vi "PWM Waveform Generator.vi"(4 "Compare Output Mode":fxp<+,2,2> format="%02b", 5 "Enable In":bool, 6 "Waveform Generation Mode":fxp<+,2,2> format="%02b", 7 "Counter is Output Compare?":bool, 10 "Counter is Min?":bool, 11 "Counter is Max?":bool) -> (3 "Output":bool)   [LabVIEW 2013]
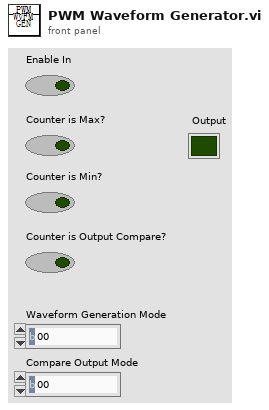
[diagram p1: front panel]
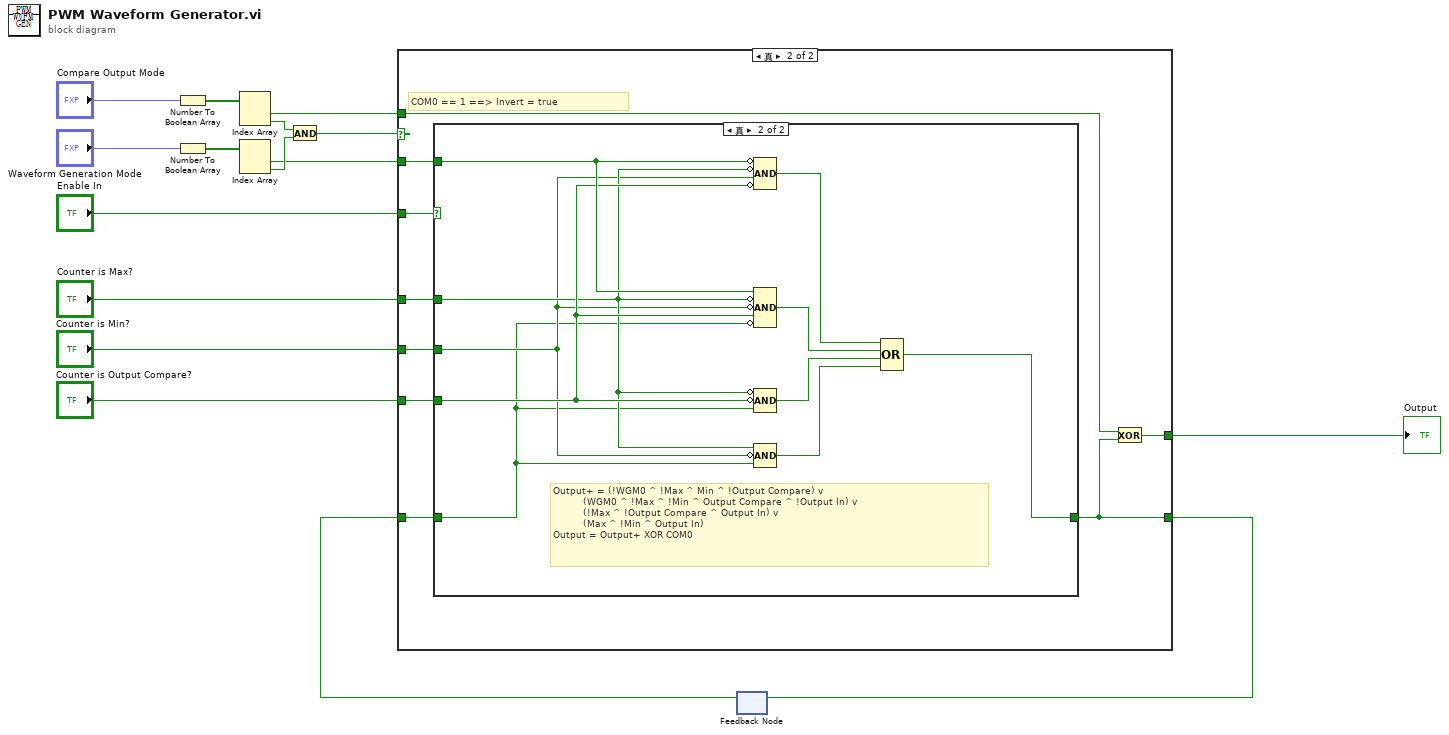
[diagram p0: block diagram]
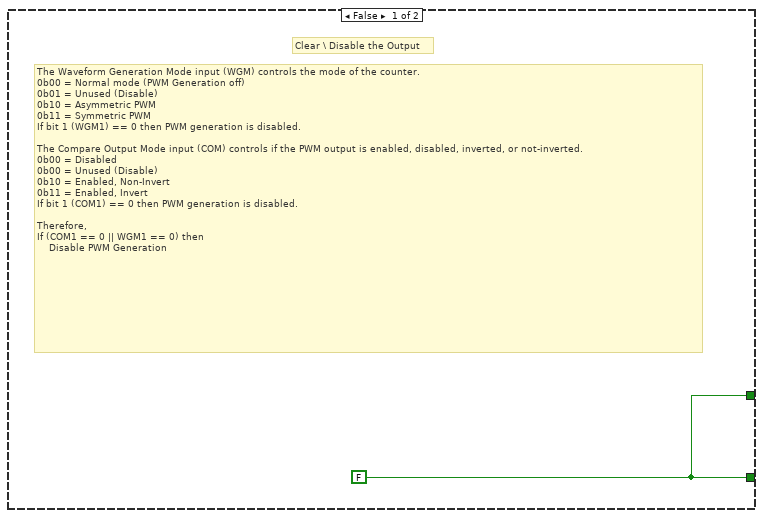
[diagram p2: hidden frame]
diagram:
  n1 = Number To Boolean Array(number="Compare Output Mode") -> (Boolean array=w15:bool[])
  n2 = Number To Boolean Array(number="Waveform Generation Mode") -> (Boolean array=w11:bool[])
  n3 = Index Array(array=w15) -> (element #1=w6:bool, element #2=w7:bool)  [unwired: 2 in]
  n4 = Index Array(array=w11) -> (element #1=w5:bool, element #2=w8:bool)  [unwired: 2 in]
  n5 = And(x=w7, y=w8) -> (x .and. y?=w9:bool)
  n6 = feedback #1() -> (w13:bool)  [unwired: 1 in]
  n7 = case shown="真" w9 {
    tunnel: "Enable In" -> [_ w26]
    tunnel: w13 -> [_ w25]
    tunnel: [w17 w18] -> w12
    tunnel: w6 -> [_ w19]
    tunnel: w5 -> [_ w24]
    tunnel: "Counter is Max?" -> [_ w23]
    tunnel: "Counter is Min?" -> [_ w22]
    tunnel: "Counter is Output Compare?" -> [_ w21]
    tunnel: [w17 w20] -> w1
    frame False {
      w17 = FALSE ("Counter is Output Compare?")
      # "The Waveform Generation Mode input (WGM) controls the mode of the counter.\n0b00 = Normal mode (PWM Generation off)\n0b01 = Unused (Disable)\n0b10 = Asymmetric PWM\n0b11 = Symmetric PWM\nIf bit 1 (WGM1) == 0 then PWM generation is disabled. \n\nThe Compare Output Mode input (COM) controls if the PWM output is enabled, disabled, inverted, or not-inverted.\n0b00 = Disabled\n0b00 = Unused (Disable)\n0b10 = Enabled, Non-Invert\n0b11 = Enabled, Invert\nIf bit 1 (COM1) == 0 then PWM generation is disabled. \n\nTherefore,\nIf (COM1 == 0 || WGM1 == 0) then\n    Disable PWM Generation"
      # "Clear \\ Disable the Output"
    }
    frame True {
      # "COM0 == 1 ==> Invert = true"
      n8 = case shown="真" w26 {
        tunnel: w25 -> [w27 w33]
        tunnel: [w27 w32] -> w18
        tunnel: w24 -> [_ w37]
        tunnel: w23 -> [_ w35]
        tunnel: w22 -> [_ w34]
        tunnel: w21 -> [_ w36]
        frame False {
          # "Hold output"
        }
        frame True {
          # "Output+ = (!WGM0 ^ !Max ^ Min ^ !Output Compare) v\n          (WGM0 ^ !Max ^ !Min ^ Output Compare ^ !Output In) v\n          (!Max ^ !Output Compare ^ Output In) v\n          (Max ^ !Min ^ Output In)\nOutput = Output+ XOR COM0"
          n9 = Compound Arithmetic op=AND(invert w37, invert w35, w34, invert w36) -> (w31:bool)
          n10 = Compound Arithmetic op=AND(w37, invert w35, invert w34, w36, invert w33) -> (w30:bool)
          n11 = Compound Arithmetic op=AND(invert w35, invert w36, w33) -> (w29:bool)
          n12 = Compound Arithmetic op=AND(w35, invert w34, w33) -> (w28:bool)
          n13 = Compound Arithmetic op=OR(w31, w30, w29, w28) -> (w32:bool)
        }
      }
      n14 = Exclusive Or(1:w18, 2:w19) -> (0:w20:bool)
    }
  }
  "Output" <- w1
  n15 = feedback-in #1(w12) -> ()
